vi "Parent Q.vi"(11 "Module in":refnum<class "Module.lvclass">) -> (2 "Parent Q":refnum<class "MessageQ.lvclass">, 3 "Module out":refnum<class "Module.lvclass">)   [LabVIEW 2020, in "Volatus.lvlib" / "Module.lvclass"]
uses:
  Module.lvclass
  Module.lvclass/Module.ctl
  MessageQ/MessageQ.lvclass
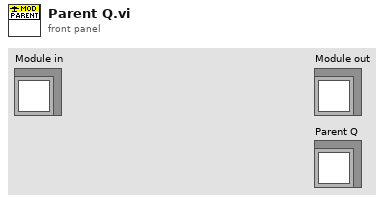
[diagram p1: front panel]
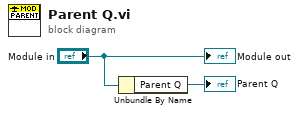
[diagram p0: block diagram]
diagram:
  n1 = Unbundle By Name("Module in") -> ("Parent Q"=→"Parent Q":refnum<class "MessageQ.lvclass">)
  "Module out" <- "Module in"
